vi "getJson.vi"(2 "error in (no error)":errorcluster caption="错误输入（无错误）", 3 "URL":string) -> (0 "error out":errorcluster caption="错误输出", 1 "响应体":string)   [LabVIEW 2012]
uses:
  <vilib>/httpClient/LabVIEWHTTPClient.lvlib
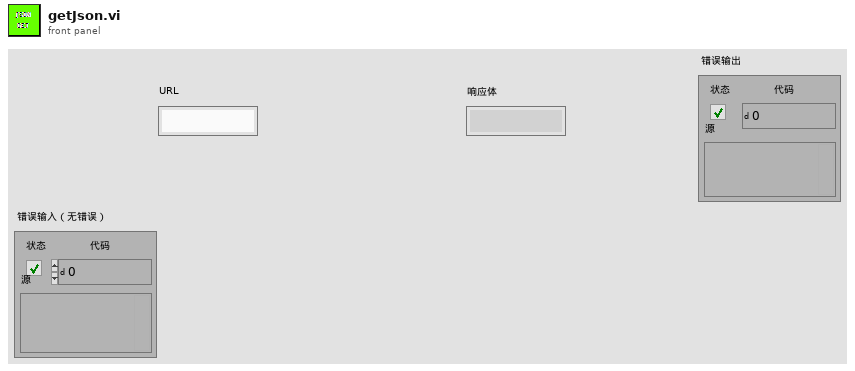
[diagram p1: front panel]
types:
  T1 = typedef "LabVIEWHTTPClient.lvlib/ClientHandle.ctl" = refnum<k1>
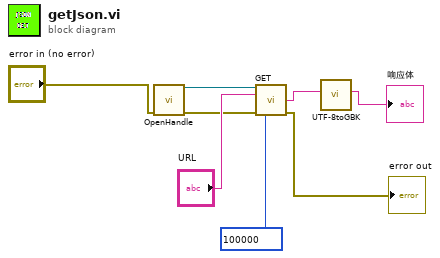
[diagram p0: block diagram]
diagram:
  n1 = call <vilib>:"OpenHandle.vi"("error in (no error)"="error in (no error)") -> ("client handle out"=w8:T1, "error out"=w6:errorcluster)  [unwired: 13 in]
  n2 = call <vilib>:"GET.vi"("client handle"=w8, "url"="URL", "error in (no error)"=w6, "timeout (10000)"=100000) -> ("body"=w4:string, "error out"=→"error out":errorcluster)  [unwired: 8 in, 2 out]
  n3 = call "UTF-8toGBK.vi"("UTF-8"=w4) -> ("GBK"=→"响应体":string)  [unwired: 10 in]
